vi "DOS Decomp for CdTe.vi"() -> ()   [LabVIEW 2010]
panel:
  out "DOS PLot":cluster{dbl[], dbl[]}[](graph)
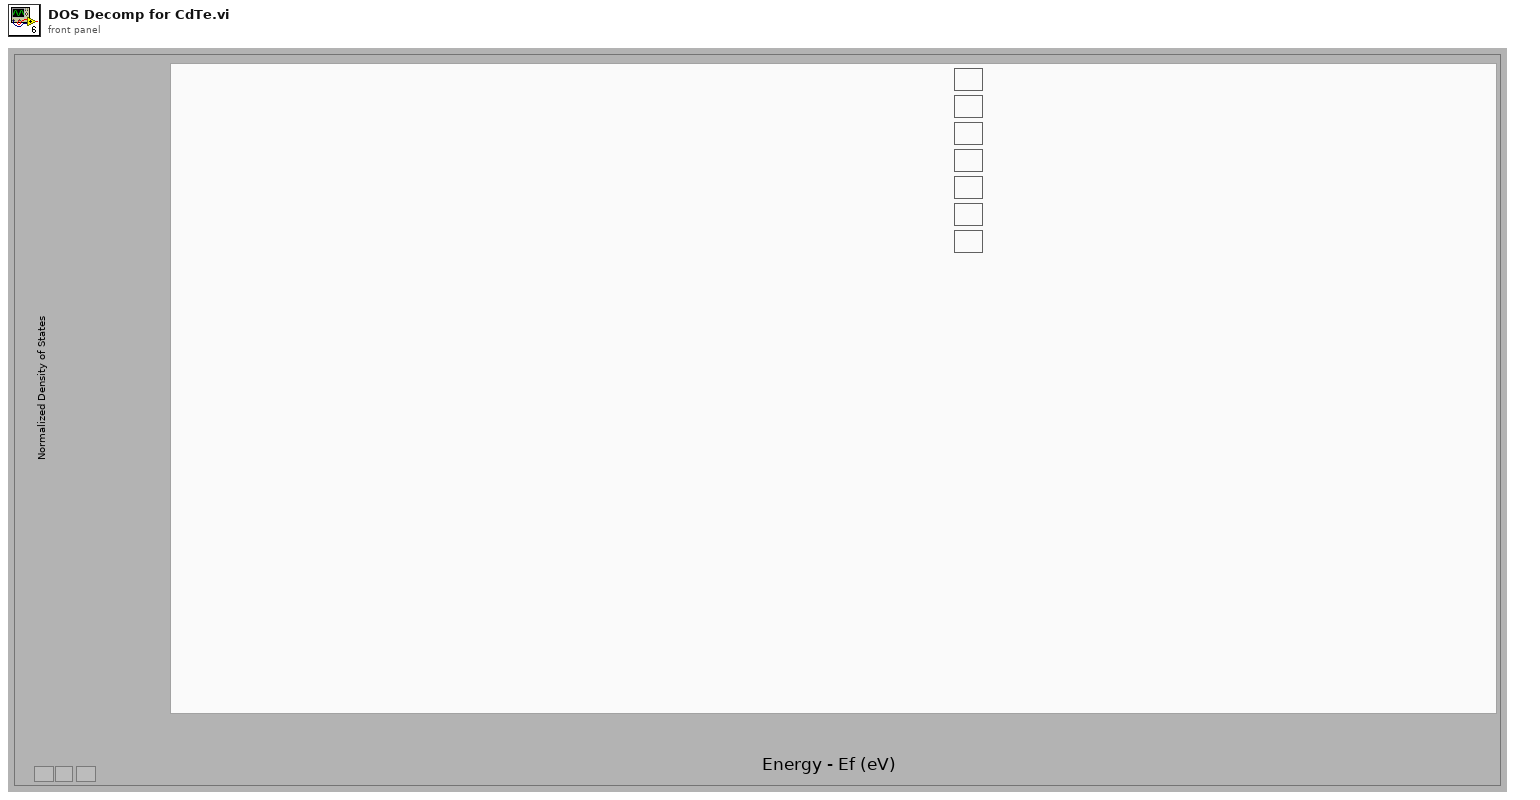
[diagram p1: front panel]
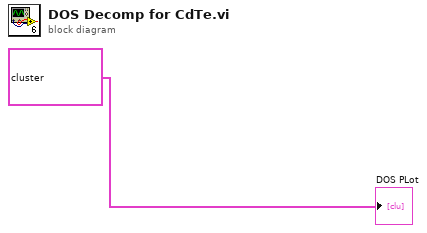
[diagram p0: block diagram]
diagram:
  "DOS PLot" <- cluster{dbl[], dbl[]}[] [{array[2000 elements], array[2000 elements]}, {array[2000 elements], array[2000 elements]}, {array[2000 elements], array[2000 elements]}, {array[2000 elements], array[2000 elements]}, {array[2000 elements], array[2000 elements]}, {array[2000 elements], array[2000 elements]}, {array[2000 elements], array[2000 elements]}] ("DOS PLot")
